vi "Get Key Values from Session.vi"(9 "Key":string, 10 "Session":string, 11 "Ini File":T1(array[cluster])) -> (1 "Number of Keys":i32, 2 "Search Key Value":u32, 3 "Keys Values in Session":cluster{"Key":string, "value":u32}[](array[cluster]))   [LabVIEW 2021]
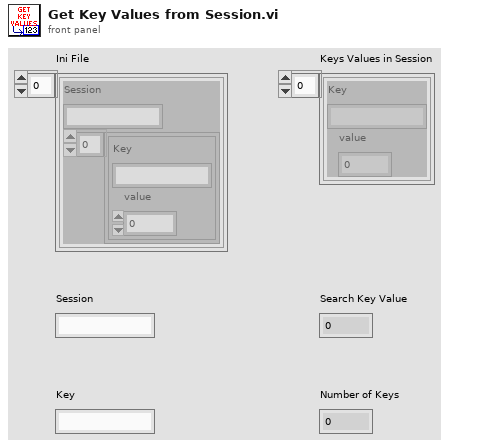
[diagram p1: front panel]
types:
  T1 = cluster{"Session":string, cluster{"Key":string, "value":u32}[]}[]
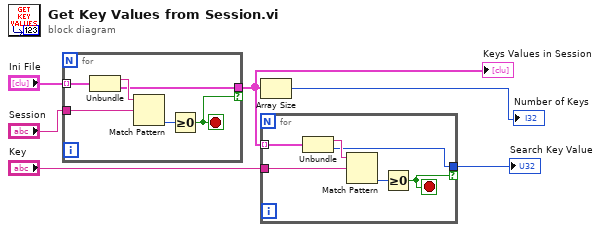
[diagram p0: block diagram]
diagram:
  n1 = for {
    tunnel: "Ini File" -> [w12] mode=indexing
    tunnel: "Session" -> [w10]
    tunnel: [w9] -> w5 if=w7
    stop <- w7 stop-if-true
    n2 = Unbundle(w12) -> ("Session"=w11:string, w9:cluster{"Key":string, "value":u32}[])
    n3 = Match Pattern(string=w11, regular expression=w10) -> (offset past match=w8:i32)  [unwired: 1 in, 3 out]
    n4 = Greater Or Equal To 0?(x=w8) -> (x >= 0?=w7:bool)
  }
  "Keys Values in Session" <- w5
  n5 = Array Size(array=w5) -> (size(s)=→"Number of Keys":i32)
  n6 = for {
    tunnel: w5 -> [w18] mode=indexing
    tunnel: "Key" -> [w16]
    tunnel: [w15] -> w4 if=w13
    stop <- w13 stop-if-true
    n7 = Unbundle(w18) -> ("Key"=w17:string, "value"=w15:u32)
    n8 = Match Pattern(string=w17, regular expression=w16) -> (offset past match=w14:i32)  [unwired: 1 in, 3 out]
    n9 = Greater Or Equal To 0?(x=w14) -> (x >= 0?=w13:bool)
  }
  "Search Key Value" <- w4
